vi "Utilities.Sizeof.Array.vi"(10 "count":i64, 11 "data type":T1) -> (3 "size":u64)   [LabVIEW 2016, in "VeriStand Data.lvlib"]
doc: "Provides the size in bytes of an array of length <B>count</B> for a specified <B>data type</B>."
uses:
  VeriStand Data.lvlib
  Typedefs/Typedefs.Data Types.ctl
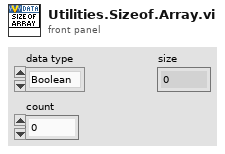
[diagram p1: front panel]
types:
  T1 = typedef "VeriStand Data.lvlib/Typedefs.Data Types.ctl" = enum16{"Boolean", "Single", "Double", "I8", "I16", "I32", "I64", "U8", "U16", "U32", "U64"}
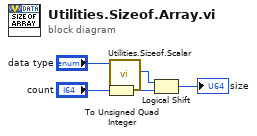
[diagram p0: block diagram]
diagram:
  n1 = To Unsigned Quad Integer(1:"count") -> (0:w1:u64)
  n2 = call "Utilities.Sizeof.Scalar.vi"("data type"="data type") -> ("bitshift count"=w3:u8)  [unwired: 9 in, 1 out]
  n3 = Logical Shift(y=w3, x=w1) -> (x << y=→"size":u64)
